vi "Manual Climb Loop.vi"   [LabVIEW 2015]
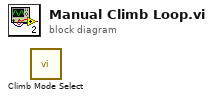
[diagram p0: block diagram]
diagram:
  n1 = call "Climb Mode Select.vi"() -> ()  [unwired: 8 in, 4 out]
